vi "Convert Data to Cartesian.vi"(10 "angle units":T1, 11 "data":T3) -> (3 "cartesian data":T2)   [LabVIEW 2017, in "NI_Robotics_2D Rangefinder Picture.lvlib"]
uses:
  <vilib>/robotics/Controls/2D Rangefinder/2D Rangefinder Picture/NI_Robotics_2D Rangefinder Picture.lvlib
  <vilib>/robotics/Controls/2D Rangefinder/2D Rangefinder Picture/Rangefinder Data.ctl
  <vilib>/robotics/Controls/2D Rangefinder/2D Rangefinder Picture/Cartesian Data.ctl
  <vilib>/robotics/Controls/Utilities/Angle Units.ctl
  <vilib>/Utility/AngleManip/Degrees to Radians (Array DBL).vi
  <vilib>/Utility/AngleManip/NI_AngleManipulation.lvlib
  <vilib>/robotics/Controls/Utilities/NI_Robotics_Control Utilities.lvlib
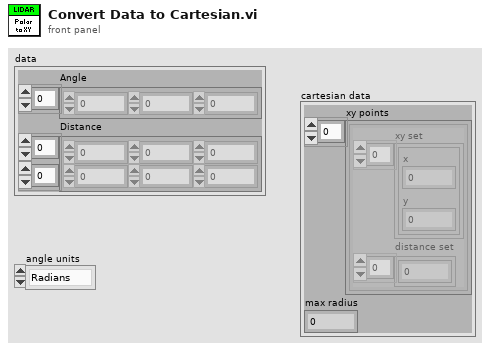
[diagram p1: front panel]
types:
  T1 = typedef "NI_Robotics_Control Utilities.lvlib/Angle Units.ctl" = enum16{"Radians", "Degrees"}
  T2 = typedef "NI_Robotics_2D Rangefinder Picture.lvlib/Cartesian Data.ctl" = cluster{"xy points":cluster{"xy set":cluster{"x":dbl, "y":dbl}[], "distance set":dbl[]}[], "max radius":dbl}
  T3 = typedef "NI_Robotics_2D Rangefinder Picture.lvlib/Rangefinder Data.ctl" = cluster{"Angle":dbl[], "Distance":dbl[][]}
  T4 = cluster{cluster{"x":dbl, "y":dbl}[], "Distance":dbl[]}
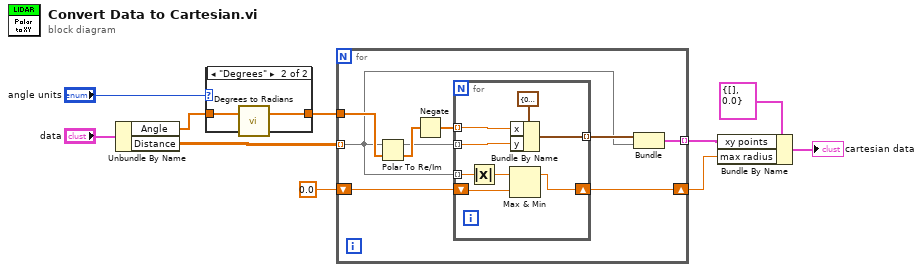
[diagram p0: block diagram]
diagram:
  n1 = Unbundle By Name("data") -> ("Angle"=w4:dbl[], "Distance"=w9:dbl[][])
  n2 = case shown="\"Degrees\"" "angle units" {
    tunnel: w4 -> [w11 w13]
    tunnel: [w11 w12] -> w3
    frame "Radians", Default {
    }
    frame "Degrees" {
      n3 = call-poly <vilib>:"Degrees to Radians.vi"("angles (deg)"=w13) -> ("angles (rad)"=w12:dbl[])  [unwired: 2 in]
    }
  }
  n4 = for {
    tunnel: w3 -> [w15]
    tunnel: w9 -> [w14] mode=indexing
    tunnel: [w18] -> w6 mode=indexing
    shift-right: [w16] -> w1
    shift-left: 0.0 -> [w17]
    n5 = Polar To Re/Im(2:w15, 3:w14) -> (0:w22:dbl[], 1:w20:dbl[])
    n6 = Negate(x=w22) -> (-x=w21:dbl[])
    n7 = for {
      tunnel: w21 -> [w28] mode=indexing
      tunnel: w20 -> [w27] mode=indexing
      tunnel: [w29] -> w19 mode=indexing
      shift-right: [w24] -> w16
      shift-left: w17 -> [w26]
      tunnel: w14 -> [w25] mode=indexing
      n8 = Absolute Value(x=w25) -> (abs(x)=w23:dbl)
      n9 = Max & Min(x=w23, y=w26) -> (max(x,y)=w24:dbl)  [unwired: 1 out]
      n10 = Bundle By Name(cluster=cluster{"x":dbl, "y":dbl} {"x"=0.0, "y"=0.0}, "x"=w28, "y"=w27) -> (w29:cluster{"x":dbl, "y":dbl})
    }
    n11 = Bundle(w19, "Distance"=w14) -> (w18:T4)  [unwired: 1 in]
  }
  n12 = Bundle By Name(cluster=T2 {"xy points"=[], "max radius"=0.0} ("cartesian data"), "xy points"=w6, "max radius"=w1) -> (→"cartesian data":T2)
